vi "Begin.vi"(8 "error in":errorcluster) -> (0 "error out":errorcluster)   [LabVIEW 2014]
doc: "Called before other user functions, this VI is expected to open initial I/O refnums, load in file data, and do all program initialization. Notice that the <B>error out</B> terminal is simply used for data flow. Wiring it to other structures or subVIs ensures that this VI runs first."
uses:
  <vilib>/Rock Robotics/WPI/DriverStation/WPI_DriverStationRobotMode2.ctl
  <vilib>/Rock Robotics/WPI/Joystick/WPI_JoystickDeviceEnum.ctl
  <vilib>/Rock Robotics/WPI/Solenoid/WPI_SolenoidChannel.ctl
  <vilib>/Rock Robotics/SystemInterfaces/DIO/FPGA_DIOPWMChannel.ctl
  <vilib>/Rock Robotics/SystemInterfaces/DIO/FPGA_DIOChannel.ctl
  <vilib>/Rock Robotics/SystemInterfaces/AI/FPGA_AIChannel.ctl
  <vilib>/Rock Robotics/SystemInterfaces/AI/FPGA_AIGyroChannel.ctl
  Robot Global Data.vi
  <vilib>/Rock Robotics/Network Tables/SD Write String Array.vi
  <vilib>/Rock Robotics/WPI/Solenoid/WPI_SolenoidOpenDouble.vi
  <vilib>/Rock Robotics/WPI/MotorControl/WPI_MotorControlOpen Talon.vi
  <vilib>/Rock Robotics/WPI/Counter/WPI_CounterDigitalInputToDigitalSource.vi
  <vilib>/Rock Robotics/WPI/Switch/WPI_SwitchOpenLimit.vi
  <vilib>/Rock Robotics/WPI/MotorControl/WPI_MotorControlOpenCANTalonSRX.vi
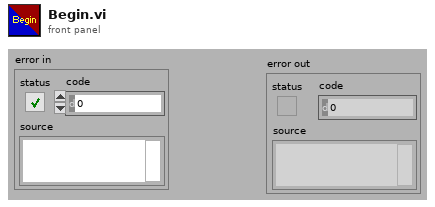
[diagram p1: front panel]
types:
  T1 = typedef "FPGA_AIGyroChannel.ctl" = enum8{"AI 0", "AI 1", "Invalid"}
  T2 = typedef "FPGA_AIChannel.ctl" = enum8{"AI 0", "AI 1", "AI 2", "AI 3", "AI MXP 0", "AI MXP 1", "AI MXP 2", "AI MXP 3", "Invalid"}
  T3 = typedef "FPGA_DIOChannel.ctl" = enum8{"DIO 0", "DIO 1", "DIO 2", "DIO 3", "DIO 4", "DIO 5", "DIO 6", "DIO 7", "DIO 8", "DIO 9", "DIO MXP 0", "DIO MXP 1", "DIO MXP 2", "DIO MXP 3", "DIO MXP 4", "DIO MXP 5", "DIO MXP 6", "DIO MXP 7", "DIO MXP 8", "DIO MXP 9", "DIO MXP 10", "DIO MXP 11", "DIO MXP 12", "DIO MXP 13", "DIO MXP 14", "DIO MXP 15", "Invalid"}
  T4 = typedef "FPGA_DIOPWMChannel.ctl" = enum8{"PWM 0", "PWM 1", "PWM 2", "PWM 3", "PWM 4", "PWM 5", "PWM 6", "PWM 7", "PWM 8", "PWM 9", "PWM MXP 0", "PWM MXP 1", "PWM MXP 2", "PWM MXP 3", "PWM MXP 4", "PWM MXP 5", "PWM MXP 6", "PWM MXP 7", "PWM MXP 8", "PWM MXP 9", "Invalid"}
  T5 = typedef "WPI_SolenoidChannel.ctl" = enum8{"Solenoid 0", "Solenoid 1", "Solenoid 2", "Solenoid 3", "Solenoid 4", "Solenoid 5", "Solenoid 6", "Solenoid 7", "Invalid"}
  T6 = typedef "WPI_JoystickDeviceEnum.ctl" = enum16{"USB 0", "USB 1", "USB 2", "USB 3", "USB 4", "USB 5"}
  T7 = typedef "WPI_DriverStationRobotMode2.ctl" = enum16{"Autonomous Disabled", "Autonomous Enabled", "Teleop Disabled", "Teleop Enabled", "Disconnected", "Finish", "Test Disabled", "Test Enabled", "Emergency Stopped"}
  T8 = typedef "WPI_MotorControlDeviceRef.ctl" = cluster{"DeviceStatus":errorcluster, "Type":T9, "PWM":cluster{"Controller":T10, "PWM Channel":T4, "DeadBand":T11}, "CAN":cluster{"Device Number":u8, "Control Mode":T12, "Semaphore":T13, "Max Vout":dbl, "TalonSRX Control Mode":T14}, "Invert":bool, "TransformRef":T15, "InvTransformRef":T15}
  T9 = typedef "WPI_MotorControlType.ctl" = enum16{"PWM", "CAN", "CANTalonSRX"}
  T10 = typedef "FPGA_TypedefDigitalModule.ctl" = enum16{"Controller 1"}
  T11 = typedef "WPI_PWMDeadband.ctl" = cluster{"Name":string, "maxPositivePwm":i32, "minPositivePwm":i32, "centerPwm":i32, "maxNegativePwm":i32, "minNegativePwm":i32, "angularRange":u16}
  T12 = typedef "WPI_CANJaguar_ControlMode.ctl" = enum8{"Percent VBus", "Current", "Speed", "Position", "Voltage"}
  T13 = typedef "Semaphore RefNum" = refnum<k1>
  T14 = typedef "WPI_CANTalonSRX_APIControlMode.ctl" = enum8{"Percent VBus", "Speed", "Position", "Slave", "Unchanged / Invalid"}
  T15 = typedef "WPI_PWMTransform_ConPane.ctl" = refnum<vi>
  T16 = typedef "WPI_JoystickDevRef.ctl" = cluster{"Device":T6}
  T17 = typedef "WPI_SolenoidDevRef.ctl" = cluster{"DevStatus":errorcluster, "Pneumatics Control Module":u8, "Forward Solenoid Channel":T5, "Reverse Solenoid Channel":T5}
  T18 = typedef "WPI_SwitchDevRef.ctl" = cluster{"DevStatus":errorcluster, "DIO Channel":T3, "Controller":T10, "CntIndex":T19, "Normally Closed":bool}
  T19 = typedef "FPGA_CounterCtrSystemIndex.ctl" = enum8{"Ctr 0", "Ctr 1", "Ctr 2", "Ctr 3", "Ctr 4", "Ctr 5", "Ctr 6", "Ctr 7", "Invalid"}
  T20 = typedef "WPI_GyroDevRef.ctl" = cluster{"DevStatus":errorcluster, "Analog Module":T21, "Analog Channel":T2, "Offset":dbl, "Gain (VoltsPerDegree/Second)":dbl}
  T21 = typedef "FPGA_TypedefAnalogModule.ctl" = enum16{"Controller 1"}
  T22 = typedef "WPI_PotentiometerDevRef.ctl" = cluster{"DevStatus":errorcluster, "Controller":T21, "Analog Channel":T2, "Invert Output":bool}
  T23 = typedef "WPI_DigitalInputDevRef.ctl" = cluster{"DevStatus":errorcluster, "DIO Channel":T3, "Controller":T10}
  T24 = typedef "FPGA_CounterEncoderSourceConvertionLVSourceType.ctl" = cluster{"DevStatus":errorcluster, "AnalogTriggerMode?":bool, "DigitalMode":cluster{"Controller":T10, "DIO Channel":T25}, "AnalogTriggerMode":cluster{"AnalogTriggerIndex":T26, "OutputType":T27}}
  T25 = typedef "FPGA_DIODigitalSourceChannel.ctl" = enum8{"DIO 0", "DIO 1", "DIO 2", "DIO 3", "DIO 4", "DIO 5", "DIO 6", "DIO 7", "DIO 8", "DIO 9", "DIO MXP 0", "DIO MXP 1", "DIO MXP 2", "DIO MXP 3", "DIO MXP 4", "DIO MXP 5", "DIO MXP 6", "DIO MXP 7", "DIO MXP 8", "DIO MXP 9", "DIO MXP 10", "DIO MXP 11", "DIO MXP 12", "DIO MXP 13", "DIO MXP 14", "DIO MXP 15", "Disabled"}
  T26 = typedef "FPGA_AnalogTriggerIndex.ctl" = enum8{"Trig 0", "Trig 1", "Trig 2", "Trig 3", "Trig 4", "Trig 5", "Trig 6", "Trig 7", "Invalid"}
  T27 = typedef "FPGA_AnalogTriggerOutType.ctl" = enum16{"InWindow", "TriggerState", "Rising", "Falling"}
  T28 = typedef "WPI_EncoderDevRef.ctl" = cluster{"DevStatus":errorcluster, "EncoderIndex":T29, "CounterIndex":T19, "DistancePerCount":dbl, "Decoding Type":T30}
  T29 = typedef "FPGA_EncoderIdx.ctl" = enum8{"Enc 0", "Enc 1", "Enc 2", "Enc 3", "Enc 4", "Enc 5", "Enc 6", "Enc 7", "Invalid"}
  T30 = typedef "WPI_EncoderType.ctl" = enum16{"1x", "2x", "4x"}
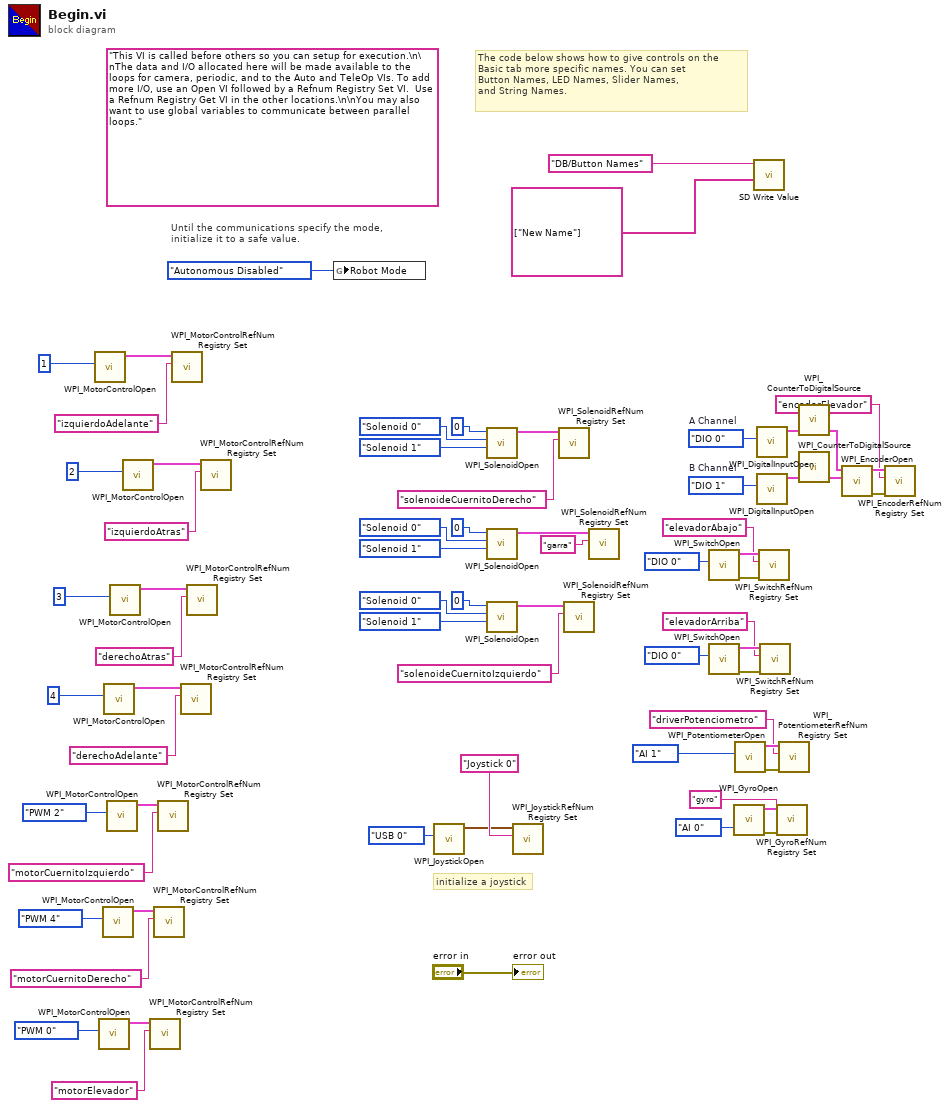
[diagram p0: block diagram]
diagram:
  w32 = FPGA_DIOChannel."DIO 1"  # B Channel
  w31 = FPGA_DIOChannel."DIO 0"  # A Channel
  (unwired) "This VI is called before others so you can setup for execution.\n\nThe data and I/O allocated here will be made available to the loops for camera, periodic, and to the Auto and TeleOp VIs. To add more I/O, use an Open VI followed by a Refnum Registry Set VI.  Use a Refnum Registry Get VI in the other locations.\n\nYou may also want to use global variables to communicate between parallel loops."
  # "The code below shows how to give controls on the\nBasic tab more specific names. You can set\nButton Names, LED Names, Slider Names,\nand String Names."
  # "initialize a joystick"
  # "Until the communications specify the mode,\ninitialize it to a safe value."
  n1 = call-poly <vilib>:"WPI_MotorControlOpen.vi"("Device Number"=u8 1) -> ("MotorControlDeviceRef"=w57:T8)  [unwired: 9 in, 1 out]
  n2 = call-poly <vilib>:"WPI_MotorControlOpen.vi"("PWM Channel"=FPGA_DIOPWMChannel."PWM 0") -> ("MotorControlDeviceRef"=w23:T8)  [unwired: 9 in, 1 out]
  n3 = call-poly <vilib>:"WPI_MotorControlOpen.vi"("PWM Channel"=FPGA_DIOPWMChannel."PWM 4") -> ("MotorControlDeviceRef"=w35:T8)  [unwired: 9 in, 1 out]
  n4 = call-poly <vilib>:"WPI_MotorControlOpen.vi"("Device Number"=u8 4) -> ("MotorControlDeviceRef"=w55:T8)  [unwired: 9 in, 1 out]
  n5 = call-poly <vilib>:"WPI_MotorControlOpen.vi"("PWM Channel"=FPGA_DIOPWMChannel."PWM 2") -> ("MotorControlDeviceRef"=w38:T8)  [unwired: 9 in, 1 out]
  n6 = call-poly <vilib>:"WPI_MotorControlOpen.vi"("Device Number"=u8 3) -> ("MotorControlDeviceRef"=w54:T8)  [unwired: 9 in, 1 out]
  n7 = call-poly <vilib>:"WPI_MotorControlOpen.vi"("Device Number"=u8 2) -> ("MotorControlDeviceRef"=w56:T8)  [unwired: 9 in, 1 out]
  n8 = call <vilib>:"WPI_MotorControlRefNum Registry Set.vi"("refnum name"="motorElevador", "MotorControlDevRef"=w23) -> ()  [unwired: 8 in, 2 out]
  n9 = call <vilib>:"WPI_MotorControlRefNum Registry Set.vi"("refnum name"="motorCuernitoDerecho", "MotorControlDevRef"=w35) -> ()  [unwired: 8 in, 2 out]
  n10 = call <vilib>:"WPI_MotorControlRefNum Registry Set.vi"("refnum name"="motorCuernitoIzquierdo", "MotorControlDevRef"=w38) -> ()  [unwired: 8 in, 2 out]
  n11 = call <vilib>:"WPI_MotorControlRefNum Registry Set.vi"("refnum name"="izquierdoAdelante", "MotorControlDevRef"=w57) -> ()  [unwired: 8 in, 2 out]
  n12 = call <vilib>:"WPI_MotorControlRefNum Registry Set.vi"("refnum name"="derechoAdelante", "MotorControlDevRef"=w55) -> ()  [unwired: 8 in, 2 out]
  n13 = call <vilib>:"WPI_MotorControlRefNum Registry Set.vi"("refnum name"="derechoAtras", "MotorControlDevRef"=w54) -> ()  [unwired: 8 in, 2 out]
  n14 = call <vilib>:"WPI_MotorControlRefNum Registry Set.vi"("refnum name"="izquierdoAtras", "MotorControlDevRef"=w56) -> ()  [unwired: 8 in, 2 out]
  n15 = global write "Robot Global Data.vi" "Robot Mode"(WPI_DriverStationRobotMode2."Autonomous Disabled" ("Robot Mode")) -> ()
  n16 = call <vilib>:"WPI_JoystickOpen.vi"("JoystickDevice"=WPI_JoystickDeviceEnum."USB 0") -> ("JoystickDevRef"=w66:T16)  [unwired: 10 in]
  n17 = call-poly <vilib>:"WPI_SolenoidOpen.vi"("Reverse Solenoid Channel"=WPI_SolenoidChannel."Solenoid 1", "Forward Solenoid Channel"=WPI_SolenoidChannel."Solenoid 0", "Pneumatics Control Module (0)"=u8 0) -> ("SolenoidDevRef"=w51:T17)  [unwired: 7 in, 1 out]
  n18 = call-poly <vilib>:"WPI_SolenoidOpen.vi"("Reverse Solenoid Channel"=WPI_SolenoidChannel."Solenoid 1", "Forward Solenoid Channel"=WPI_SolenoidChannel."Solenoid 0", "Pneumatics Control Module (0)"=u8 0) -> ("SolenoidDevRef"=w53:T17)  [unwired: 7 in, 1 out]
  n19 = call-poly <vilib>:"WPI_SolenoidOpen.vi"("Reverse Solenoid Channel"=WPI_SolenoidChannel."Solenoid 1", "Forward Solenoid Channel"=WPI_SolenoidChannel."Solenoid 0", "Pneumatics Control Module (0)"=u8 0) -> ("SolenoidDevRef"=w52:T17)  [unwired: 7 in, 1 out]
  n20 = call <vilib>:"WPI_JoystickRefNum Registry Set.vi"("refnum name"="Joystick 0", "JoystickDevRef"=w66) -> ()  [unwired: 8 in, 2 out]
  n21 = call <vilib>:"WPI_SolenoidRefNum Registry Set.vi"("refnum name"="solenoideCuernitoDerecho", "SolenoidDevRef"=w51) -> ()  [unwired: 8 in, 2 out]
  n22 = call <vilib>:"WPI_SolenoidRefNum Registry Set.vi"("refnum name"="solenoideCuernitoIzquierdo", "SolenoidDevRef"=w52) -> ()  [unwired: 8 in, 2 out]
  n23 = call <vilib>:"WPI_SolenoidRefNum Registry Set.vi"("refnum name"="garra", "SolenoidDevRef"=w53) -> ()  [unwired: 8 in, 2 out]
  n24 = call-poly <vilib>:"WPI_SwitchOpen.vi"("DIO Channel"=FPGA_DIOChannel."DIO 0") -> ("error out"=w20:errorcluster, "SwitchDevRef"=w19:T18)  [unwired: 9 in]
  n25 = call-poly <vilib>:"WPI_SwitchOpen.vi"("DIO Channel"=FPGA_DIOChannel."DIO 0") -> ("error out"=w17:errorcluster, "SwitchDevRef"=w16:T18)  [unwired: 9 in]
  n26 = call <vilib>:"WPI_GyroOpen.vi"("Analog Channel"=FPGA_AIGyroChannel."AI 0") -> ("error out"=w8:errorcluster, "GyroDevRef"=w7:T20)  [unwired: 8 in, 1 out]
  n27 = call <vilib>:"WPI_PotentiometerOpen.vi"("Analog Channel"=FPGA_AIChannel."AI 1") -> ("error out"=w12:errorcluster, "PotDevRef"=w11:T22)  [unwired: 9 in]
  n28 = call-poly <vilib>:"SD Write Value.vi"("String Array"=string[] ["New Name"], "Name"="DB/Button Names") -> ()  [unwired: 8 in, 2 out]
  n29 = call <vilib>:"WPI_DigitalInputOpen.vi"("DIO Channel"=w31) -> ("DigitalInputDevRef"=w28:T23)  [unwired: 2 in, 8 out]
  n30 = call <vilib>:"WPI_DigitalInputOpen.vi"("DIO Channel"=w32) -> ("DigitalInputDevRef"=w29:T23)  [unwired: 2 in, 8 out]
  n31 = call <vilib>:"WPI_SwitchRefNum Registry Set.vi"("error in (no error)"=w20, "refnum name"="elevadorAbajo", "SwitchDevRef"=w19) -> ()  [unwired: 7 in, 2 out]
  n32 = call <vilib>:"WPI_SwitchRefNum Registry Set.vi"("error in (no error)"=w17, "refnum name"="elevadorArriba", "SwitchDevRef"=w16) -> ()  [unwired: 7 in, 2 out]
  n33 = call <vilib>:"WPI_GyroRefNum Registry Set.vi"("error in (no error)"=w8, "refnum name"="gyro", "GyroDevRef"=w7) -> ()  [unwired: 7 in, 2 out]
  n34 = call <vilib>:"WPI_PotentiometerRefNum Registry Set.vi"("error in (no error)"=w12, "refnum name"="driverPotenciometro", "PotDevRef"=w11) -> ()  [unwired: 7 in, 2 out]
  n35 = call-poly <vilib>:"WPI_CounterToDigitalSource.vi"("DigitalInputDevRef"=w28) -> ("Digital Source"=w27:T24)  [unwired: 6 out]
  n36 = call-poly <vilib>:"WPI_CounterToDigitalSource.vi"("DigitalInputDevRef"=w29) -> ("Digital Source"=w30:T24)  [unwired: 6 out]
  n37 = call <vilib>:"WPI_EncoderOpen.vi"("BSource"=w30, "ASource"=w27) -> ("error out"=w25:errorcluster, "EncoderDevRef"=w26:T28)  [unwired: 6 in, 2 out]
  n38 = call <vilib>:"WPI_EncoderRefNum Registry Set.vi"("error in (no error)"=w25, "refnum name"="encoderElevador", "EncoderDevRef"=w26) -> ()  [unwired: 7 in, 2 out]
  "error out" <- "error in"
